vi "State History.vi"(0 "Current State in":string) -> (6 "State History":string, 7 "Current State out":string)   [LabVIEW 2016, in "Instrument.Lockin.lvclass"]
uses:
  Instrument.Lockin.lvclass
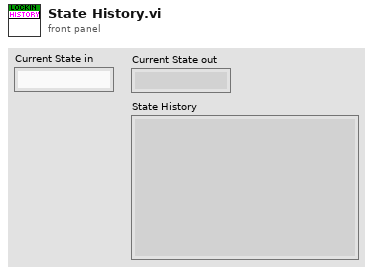
[diagram p1: front panel]
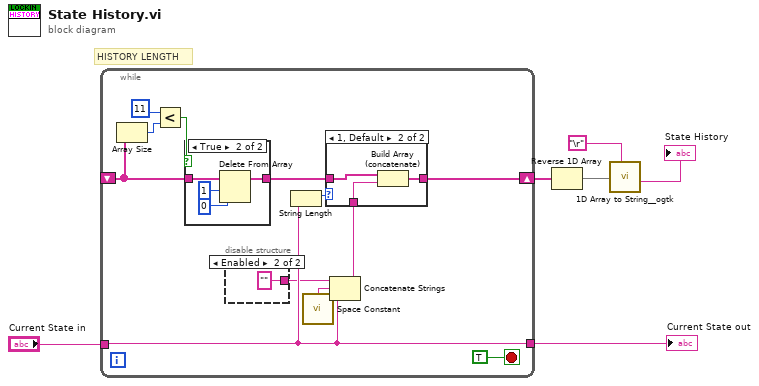
[diagram p0: block diagram]
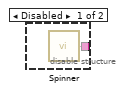
[diagram p2: hidden frame]
diagram:
  # "HISTORY LENGTH"
  n1 = while {
    tunnel: "Current State in" -> [w9]
    tunnel: [w9] -> w6
    shift-right: [w11] -> w2
    shift-left: _ -> [w12]
    stop <- TRUE stop-if-true
    n2 = Array Size(array=w12) -> (size(s)=w16:i32)
    n3 = Less?(x=11 ("length"), y=w16) -> (x < y?=w18:bool)
    n4 = case shown="True" w18 {
      tunnel: w12 -> [w25 w26]
      tunnel: [w25 w28] -> w17
      frame False {
      }
      frame True {
        n5 = Delete From Array(array=w26, length=1, index=0) -> (array with subset deleted=w28:string[])  [unwired: 1 out]
      }
    }
    n6 = disable-structure shown="Enabled" {
      disable-tunnel: [w19 "" ("Spinner Out")] -> w8
      frame Disabled {
        n7 = call "Spinner.vi"() -> ("Spinner Out"=w19:string)  [unwired: 5 in]
      }
      frame Enabled {
      }
    }
    n8 = String Length(string=w9) -> (length=w15:i32)
    n9 = call <vilib>:"Space Constant.vi"() -> ("String"=w7:string)
    n10 = Concatenate Strings(w8, w7, w9) -> (w10:string)
    n11 = case shown="1, Default" w15 {
      tunnel: w17 -> [w21 w23]
      tunnel: [w21 w24] -> w11
      tunnel: w10 -> [_ w22]
      frame 0 {
      }
      frame 1, Default {
        n12 = Build Array (concatenate)(w23, w22) -> (w24:string[])
      }
    }
  }
  "Current State out" <- w6
  n13 = Reverse 1D Array(array=w2) -> (reversed array=w1:string[])
  n14 = call <userlib>:"1D Array to String__ogtk.vi"("delimiter (Tab)"="\r", "Array of Strings"=w1) -> ("delimited string"=→"State History":string)  [unwired: 9 in]
